vi "Analysis.LevelTransition.vi"(8 "error in":errorcluster, 11 "Data":path) -> (0 "error out":errorcluster, 1 "Failed Channels":string[](array[string]), 2 "Result":bool[](array[boolean]))   [LabVIEW 2014, in "NIAnalysis.lvlib"]
uses:
  NIAnalysis.lvlib
  Analysis.SingleChannelLevelTransitionLogic.vi
  Constants.vi
panel:
  out "Fail":bool
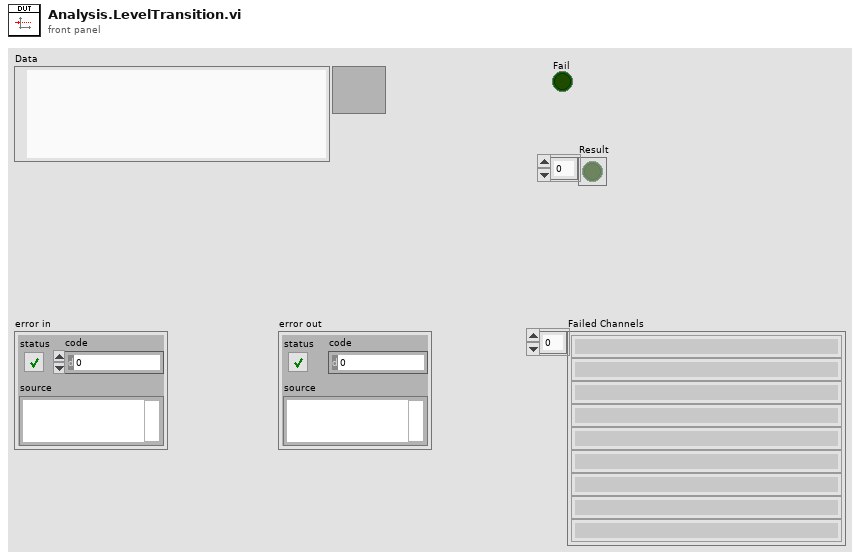
[diagram p1: front panel]
types:
  T1 = typedef "NIAnalysis.lvlib/Public.LVAnalysis.ctl" = cluster{"ODH":T2, "OPH_Duty":T2, "OPH_Freq":T2}
  T2 = typedef "NIAnalysis.lvlib/Public.ChLVAnalysis.ctl" = cluster{"Level":dbl, "Band (+-)":dbl, "TimeTolerance":dbl}
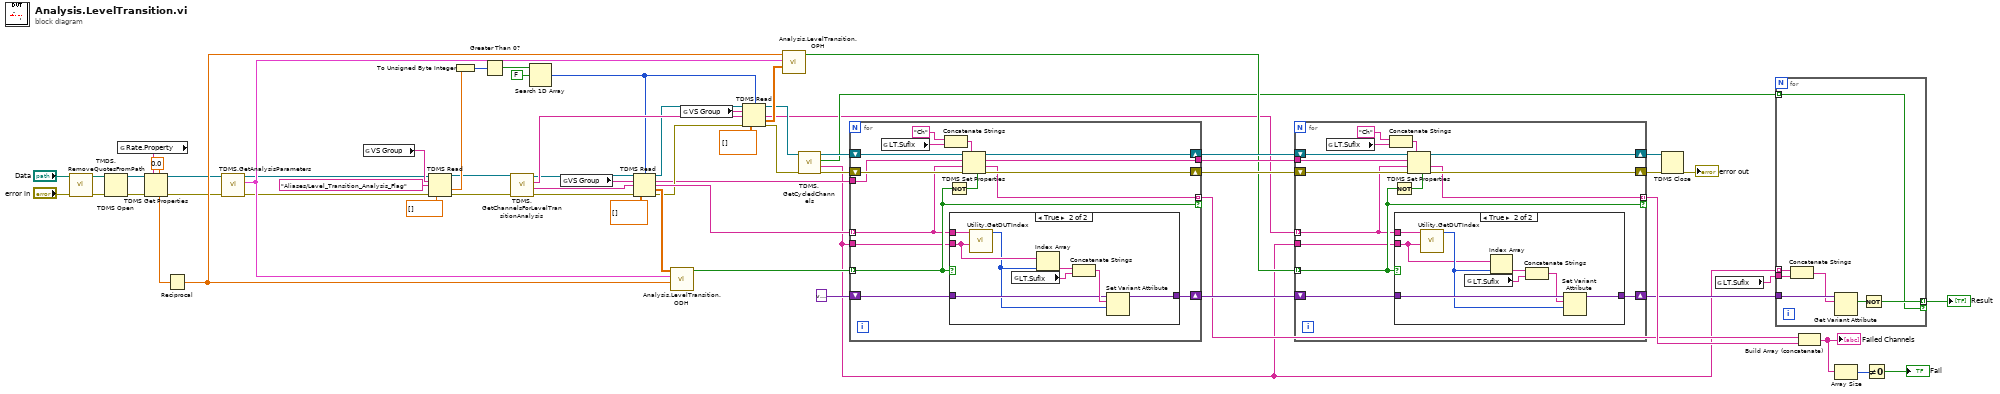
[diagram p0: block diagram]
diagram:
  n1 = call "TMDS.RemoveQuotesFromPath.vi"("error in (no error)"="error in", "Data"="Data") -> ("error out"=w2:errorcluster, "Path"=w3:path)  [unwired: 8 in]
  n2 = TDMS Open(8:w2, 11:w3) -> (0:w21:errorcluster, 3:w20:refnum<k34>)  [unwired: 5 in]
  n3 = global read "Constants.vi" "Rate.Property"() -> (w59:string)
  n4 = TDMS Get Properties(5:0.0, 7:w59, 8:w21, 11:w20) -> (0:w22:errorcluster, 3:w23:refnum<k34>, 4:w63:dbl)  [unwired: 2 in, 3 out]
  n5 = Reciprocal(x=w63) -> (1/x=w44:dbl)
  n6 = call "TDMS.GetAnalysisParameters.vi"("error in (no error)"=w22, "TDMS Ref"=w23) -> ("error out"=w25:errorcluster, "LVTransitionParameters"=w34:T1, "TDMS Ref"=w24:refnum<k34>)  [unwired: 6 in, 1 out]
  n7 = global read "Constants.vi" "VS Group"() -> (w41:string)
  n8 = TDMS Read(0:w24, 5:w41, 7:"Aliases/Level_Transition_Analysis_Flag" ("channel name(s) in"), 11:w25, 12:dbl[] []) -> (4:w26:refnum<k34>, 10:w39:dbl[], 15:w27:errorcluster)  [unwired: 3 in, 3 out]
  n9 = To Unsigned Byte Integer(number=w39) -> (unsigned 8bit integer=w38:u8[])
  n10 = Greater Than 0?(x=w38) -> (x > 0?=w37:bool[])
  n11 = call "TDMS.GetChannelsForLevelTransitionAnalysis.vi"("error in (no error)"=w27, "TDMS Ref"=w26) -> ("error out"=w33:errorcluster, "ODH Channels"=w6:string[], "OPH Channels"=w54:string[], "TDMS Ref out"=w32:refnum<k34>)  [unwired: 6 in]
  n12 = Search 1D Array(1D array=w37, element=FALSE) -> (index of element=w35:i32)  [unwired: 1 in]
  n13 = global read "Constants.vi" "VS Group"() -> (w50:string)
  n14 = TDMS Read(0:w32, 2:w35, 5:w50, 7:w6, 11:w33, 12:dbl[][] []) -> (4:w45:refnum<k34>, 6:w55:string, 8:w57:string[], 10:w58:dbl[][], 15:w56:errorcluster)  [unwired: 2 in, 1 out]
  n15 = call "Analysis.LevelTransition.ODH.vi"("Numeric"=w44, "LVTransitionParameters"=w34, "Array in"=w58) -> ("Array out"=w51:bool[])  [unwired: 8 in]
  n16 = global read "Constants.vi" "VS Group"() -> (w19:string)
  n17 = TDMS Read(0:w45, 2:w35, 5:w19, 7:w54, 11:w56, 12:dbl[][] []) -> (4:w29:refnum<k34>, 8:w12:string[], 10:w52:dbl[][], 15:w31:errorcluster)  [unwired: 2 in, 2 out]
  n18 = call "Analysis.LevelTransition.OPH.vi"("Array in"=w52, "LVTransitionParameters"=w34, "Numeric"=w44) -> ("Array out"=w14:bool[])  [unwired: 8 in]
  n19 = call "TDMS.GetCycledChannels.vi"("error in (no error)"=w31, "TDMS Ref"=w29) -> ("error out"=w30:errorcluster, "DUTs"=w5:string[], "Cycled"=w13:bool[], "TDMS Ref"=w28:refnum<k34>)  [unwired: 6 in]
  n20 = for {
    tunnel: w51 -> [w69] mode=indexing
    tunnel: w57 -> [w66] mode=indexing
    shift-right: [w74] -> w17
    shift-left: w30 -> [w77]
    shift-right: [w73] -> w18
    shift-left: w28 -> [w76]
    tunnel: [w71] -> w7 mode=indexing if=w69
    shift-right: [w67] -> w15
    shift-left: variant -> [w68]
    tunnel: w55 -> [w75]
    tunnel: [w72] -> w16
    tunnel: w5 -> [w65]
    n21 = global read "Constants.vi" "LT.Sufix"() -> (w78:string)
    n22 = Concatenate Strings("Ch" ("group name in"), w78) -> (w79:string)
    n23 = Not(x=w69) -> (.not. x?=w70:bool)
    n24 = case shown="True" w69 {
      tunnel: w68 -> [w81 w88]
      tunnel: [w81 w87] -> w67
      tunnel: w66 -> [_ w85]
      tunnel: w65 -> [_ w84]
      frame False {
      }
      frame True {
        n25 = call "Utility.GetDUTIndex.vi"("DUTs"=w84, "Channel"=w85) -> ("Index"=w82:i32)  [unwired: 8 in, 1 out]
        n26 = global read "Constants.vi" "LT.Sufix"() -> (w86:string)
        n27 = Index Array(array=w84, index=w82) -> (element=w83:string)
        n28 = Concatenate Strings(w83, w86) -> (w89:string)
        n29 = Set Variant Attribute(Variant=w88, name=w89, value=w82) -> (Variant out=w87:variant)  [unwired: 1 in, 2 out]
      }
    }
    n30 = TDMS Set Properties(5:w70, 7:w79, 8:w77, 9:w66, 10:w75, 11:w76) -> (0:w74:errorcluster, 1:w71:string, 2:w72:string, 3:w73:refnum<k34>)
  }
  n31 = for {
    tunnel: w14 -> [w94] mode=indexing
    tunnel: w12 -> [w91] mode=indexing
    shift-right: [w98] -> w8
    shift-left: w17 -> [w101]
    shift-right: [w97] -> w9
    shift-left: w18 -> [w100]
    tunnel: [w96] -> w11 mode=indexing if=w94
    shift-right: [w92] -> w10
    shift-left: w15 -> [w93]
    tunnel: w16 -> [w99]
    tunnel: w5 -> [w90]
    n32 = global read "Constants.vi" "LT.Sufix"() -> (w102:string)
    n33 = Concatenate Strings("Ch" ("group name in"), w102) -> (w103:string)
    n34 = Not(x=w94) -> (.not. x?=w95:bool)
    n35 = case shown="True" w94 {
      tunnel: w93 -> [w105 w113]
      tunnel: [w105 w112] -> w92
      tunnel: w91 -> [_ w111]
      tunnel: w90 -> [_ w107]
      frame False {
      }
      frame True {
        n36 = call "Utility.GetDUTIndex.vi"("DUTs"=w107, "Channel"=w111) -> ("Index"=w108:i32)  [unwired: 8 in, 1 out]
        n37 = global read "Constants.vi" "LT.Sufix"() -> (w110:string)
        n38 = Index Array(array=w107, index=w108) -> (element=w109:string)
        n39 = Concatenate Strings(w109, w110) -> (w106:string)
        n40 = Set Variant Attribute(Variant=w113, name=w106, value=w108) -> (Variant out=w112:variant)  [unwired: 1 in, 2 out]
      }
    }
    n41 = TDMS Set Properties(5:w95, 7:w103, 8:w101, 9:w91, 10:w99, 11:w100) -> (0:w98:errorcluster, 1:w96:string, 3:w97:refnum<k34>)  [unwired: 1 out]
  }
  n42 = TDMS Close(8:w8, 11:w9) -> (0:→"error out":errorcluster)  [unwired: 1 out]
  n43 = global read "Constants.vi" "LT.Sufix"() -> (w60:string)
  n44 = for {
    tunnel: w5 -> [w120] mode=indexing
    tunnel: w60 -> [w119]
    tunnel: w10 -> [w118]
    tunnel: [w115] -> w62 mode=indexing if=w114
    tunnel: w13 -> [w114] mode=indexing
    n45 = Concatenate Strings(w120, w119) -> (w116:string)
    n46 = Get Variant Attribute(Variant=w118, name=w116) -> (found=w117:bool)  [unwired: 2 in, 3 out]
    n47 = Not(x=w117) -> (.not. x?=w115:bool)
  }
  "Result" <- w62
  n48 = Build Array (concatenate)(w7, w11) -> (w49:string[])
  "Failed Channels" <- w49
  n49 = Array Size(array=w49) -> (size(s)=w48:i32)
  n50 = Not Equal To 0?(x=w48) -> (x != 0?=→"Fail":bool)
